vi "PSTR-Compute Response Amplitude.vi"(0 "Runtime in":T1 {"window" items=["None ", "Hanning", "Hamming", "Blackman-Harris", "Exact Blackman", "Blackman", "Flat Top", "4 Term B-Harris ", "7 Term B-Harris", "Low Sidelobe"]}, 5 "Data":dbl[](array[numeric]), 7 "On in":dbl, 11 "Out in":dbl) -> (8 "On out":dbl, 15 "Off out":dbl)   [LabVIEW 2020]
uses:
  Typedefs/PSTR-Runtime Data.ctl
  epl-vi-lib/Signal Synthesis VIs/4th Generation/Classes/SignalManager/SignalManager.lvclass
  <vilib>/Analysis/baseanly.llb/Mean (DBL).vi
  <vilib>/Analysis/NI_AALBase.lvlib
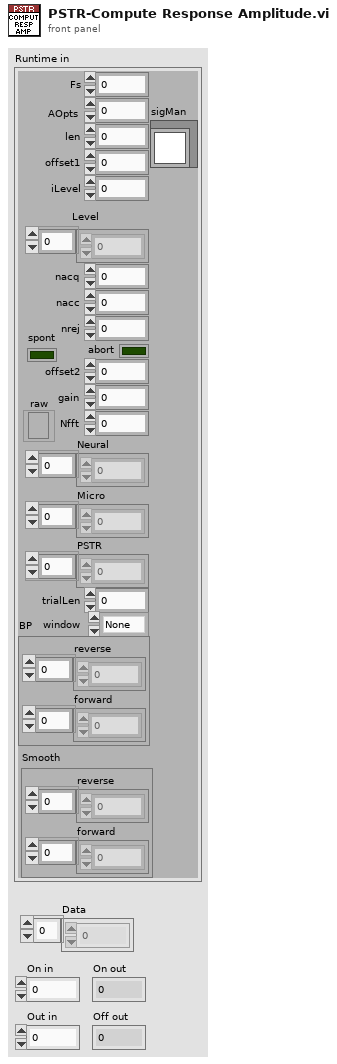
[diagram p1: front panel]
types:
  T1 = typedef "PSTR-Runtime Data.ctl" = cluster{"Fs":dbl, "AOpts":i32, "len":i32, "offset1":i32, "iLevel":i32, "Level":dbl[], "nacc":i32, "nrej":i32, "nacq":i32, "abort":bool, "offset2":i32, "gain":dbl, "Nfft":i32, "Neural":dbl[], "Micro":dbl[], "raw":refnum<file>, "spont":bool, "PSTR":dbl[], "trialLen":i32, "window":u16, "BP":cluster{"reverse":dbl[], "forward":dbl[]}, "Smooth":cluster{"reverse":dbl[], "forward":dbl[]}, "sigMan":refnum<class "SignalManager.lvclass">}
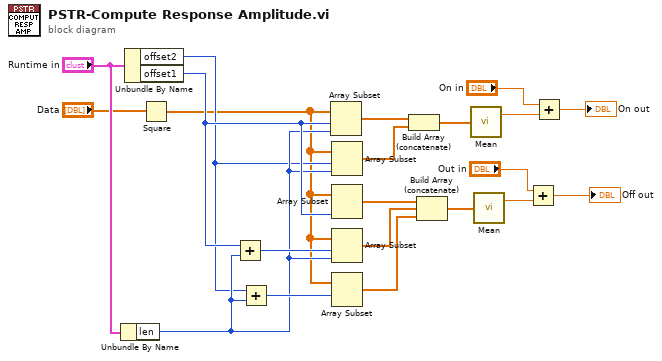
[diagram p0: block diagram]
diagram:
  n1 = Unbundle By Name("Runtime in") -> ("len"=w16:i32)
  n2 = Unbundle By Name("Runtime in") -> ("offset2"=w15:i32, "offset1"=w19:i32)
  n3 = Square(x="Data") -> (x^2=w14:dbl[])
  n4 = Add(x=w19, y=w16) -> (x+y=w18:i32)
  n5 = Add(x=w15, y=w16) -> (x+y=w17:i32)
  n6 = Array Subset(array=w14, index=w19, length=w16) -> (w13:dbl[])
  n7 = Array Subset(array=w14, index=w15, length=w16) -> (w12:dbl[])
  n8 = Array Subset(array=w14, length=w19) -> (w11:dbl[])  [unwired: 1 in]
  n9 = Array Subset(array=w14, index=w18, length=w16) -> (w10:dbl[])
  n10 = Array Subset(array=w14, index=w17) -> (w9:dbl[])  [unwired: 1 in]
  n11 = Build Array (concatenate)(w13, w12) -> (w8:dbl[])
  n12 = Build Array (concatenate)(w11, w10, w9) -> (w7:dbl[])
  n13 = call-poly <vilib>:"Mean.vi"("X"=w8) -> ("mean"=w6:dbl)  [unwired: 1 out]
  n14 = call-poly <vilib>:"Mean.vi"("X"=w7) -> ("mean"=w2:dbl)  [unwired: 1 out]
  n15 = Add(x="Out in", y=w2) -> (x+y=→"Off out":dbl)
  n16 = Add(x="On in", y=w6) -> (x+y=→"On out":dbl)
